vi "Remove Connection Record Reference.vi"(8 "error in (no error)":errorcluster, 10 "Connected?":bool, 11 "Data Value Reference in":refnum<data-value>) -> (0 "error out":errorcluster, 3 "Data Value Reference out":refnum<data-value>)   [LabVIEW 2017, in "SubVIs.lvlib" / "TCP Slave.lvclass"]
uses:
  <vilib>/Modbus/subvis/Protocol/TCP/TCP Slave/TCP Slave.lvclass
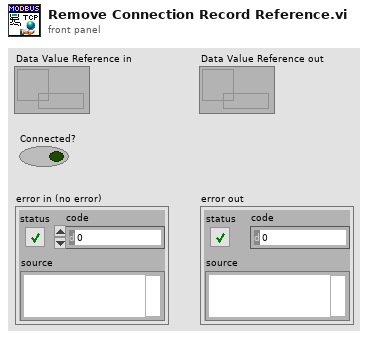
[diagram p1: front panel]
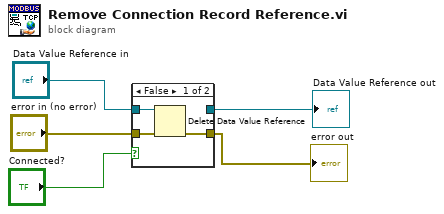
[diagram p0: block diagram]
diagram:
  n1 = case shown="False" "Connected?" {
    tunnel: "Data Value Reference in" -> [w8 w10]
    tunnel: [_ w10] -> w2
    tunnel: "error in (no error)" -> [w7 w9]
    tunnel: [w6 w9] -> w5
    frame False {
      n2 = Delete Data Value Reference(data value reference=w8, error in=w7) -> (error out=w6:errorcluster)  [unwired: 1 out]
    }
    frame True {
    }
  }
  "error out" <- w5
  "Data Value Reference out" <- w2
